vi "Block DMA.vi"(4 "RFM offset":u32 format="%.0x", 6 "Transfer Size (bytes)":u32=1024000, 7 "Wait Mode":T1, 8 "error in (no error)":errorcluster, 11 "VISA Resource Name":refnum<visa-resource-name>="PXI4::14::INSTR") -> (0 "error out":errorcluster, 1 "Read Timed Out?":bool, 2 "Write Timed Out?":bool, 3 "Success?":bool)   [LabVIEW 2017]
uses:
  niveristand-data-sharing-framework-custom-device-plugins/Components/Transceivers/GE Reflective Memory/Driver/Source/Typedefs/GE 5565PIORC.Typedef.DMA Wait Mode.ctl
  niveristand-data-sharing-framework-custom-device-plugins/Components/Transceivers/GE Reflective Memory/Driver/Source/GE 5565PIORC.lvclass/GE 5565PIORC.ctl
  niveristand-data-sharing-framework-custom-device-plugins/Components/Transceivers/GE Reflective Memory/Driver/Source/Methods/GE 5565PIORC.DMA.Block.Write (String).vi
  niveristand-data-sharing-framework-custom-device-plugins/Components/Transceivers/GE Reflective Memory/Driver/Source/Methods/GE 5565PIORC.DMA.Create Transfer (Block).vi
  niveristand-data-sharing-framework-custom-device-plugins/Components/Transceivers/GE Reflective Memory/Driver/Source/Methods/GE 5565PIORC.DMA.Get Transfer Components (Block).vi
  niveristand-data-sharing-framework-custom-device-plugins/Components/Transceivers/GE Reflective Memory/Driver/Source/Methods/GE 5565PIORC.DMA.Block.Read (String).vi
  niveristand-data-sharing-framework-custom-device-plugins/Components/Transceivers/GE Reflective Memory/Driver/Source/Properties/Registers/GE 5565PIORC.Registers.LAS1RR.PCI Address Range.Get.vi
  niveristand-data-sharing-framework-custom-device-plugins/Components/Transceivers/GE Reflective Memory/Driver/Source/Methods/GE 5565PIORC.PXI Interrupts.Enable.vi
  niveristand-data-sharing-framework-custom-device-plugins/Components/Transceivers/GE Reflective Memory/Driver/Source/Properties/Registers/GE 5565PIORC.Registers.DMACSR0.Channel 0 Enable.Set.vi
  niveristand-data-sharing-framework-custom-device-plugins/Components/Transceivers/GE Reflective Memory/Driver/Source/Properties/Registers/GE 5565PIORC.Registers.INTCSR.Local DMA Channel 0 Interrupt Enable.Set.vi
  niveristand-data-sharing-framework-custom-device-plugins/Components/Transceivers/GE Reflective Memory/Driver/Source/Properties/GE 5565PIORC.Read VISA MEMACC.vi
  niveristand-data-sharing-framework-custom-device-plugins/Components/Transceivers/GE Reflective Memory/Driver/Source/Methods/GE 5565PIORC.DMA.Create Transfer (Scatter-Gather).vi
  niveristand-data-sharing-framework-custom-device-plugins/Components/Transceivers/GE Reflective Memory/Driver/Source/Methods/GE 5565PIORC.DMA.Configure.vi
  niveristand-data-sharing-framework-custom-device-plugins/Components/Transceivers/GE Reflective Memory/Driver/Source/Methods/GE 5565PIORC.PXI Interrupts.Discard Events.vi
  niveristand-data-sharing-framework-custom-device-plugins/Components/Transceivers/GE Reflective Memory/Driver/Source/Methods/GE 5565PIORC.DMA.Start.vi
  niveristand-data-sharing-framework-custom-device-plugins/Components/Transceivers/GE Reflective Memory/Driver/Source/Methods/GE 5565PIORC.DMA.Wait for Done.vi
  niveristand-data-sharing-framework-custom-device-plugins/Components/Transceivers/GE Reflective Memory/Driver/Source/Methods/GE 5565PIORC.DMA.Block.Clear.vi
  niveristand-data-sharing-framework-custom-device-plugins/Components/Transceivers/GE Reflective Memory/Driver/Source/Methods/GE 5565PIORC.DMA.Block.Clear (multiple).vi
  niveristand-data-sharing-framework-custom-device-plugins/Components/Transceivers/GE Reflective Memory/Driver/Source/Properties/Registers/GE 5565PIORC.Registers.Local Configuration.Read.vi
  niveristand-data-sharing-framework-custom-device-plugins/Components/Transceivers/GE Reflective Memory/Driver/Source/Properties/Registers/GE 5565PIORC.Registers.Local Configuration.Read (U32).vi
  niveristand-data-sharing-framework-custom-device-plugins/Components/Transceivers/GE Reflective Memory/Driver/Source/Properties/Registers/GE 5565PIORC.Registers.Local Configuration.Read (U8).vi
  niveristand-data-sharing-framework-custom-device-plugins/Components/Transceivers/GE Reflective Memory/Driver/Source/Properties/Registers/GE 5565PIORC.Registers.Local Configuration.Write.vi
  niveristand-data-sharing-framework-custom-device-plugins/Components/Transceivers/GE Reflective Memory/Driver/Source/Properties/Registers/GE 5565PIORC.Registers.Local Configuration.Write (U8).vi
  niveristand-data-sharing-framework-custom-device-plugins/Components/Transceivers/GE Reflective Memory/Driver/Source/Methods/GE 5565PIORC.Bit Manipulation.Set Bit.vi
  niveristand-data-sharing-framework-custom-device-plugins/Components/Transceivers/GE Reflective Memory/Driver/Source/Methods/GE 5565PIORC.Bit Manipulation.Set Bit (U8).vi
  niveristand-data-sharing-framework-custom-device-plugins/Components/Transceivers/GE Reflective Memory/Driver/Source/Properties/Registers/GE 5565PIORC.Registers.Local Configuration.Write (U32).vi
  niveristand-data-sharing-framework-custom-device-plugins/Components/Transceivers/GE Reflective Memory/Driver/Source/Methods/GE 5565PIORC.Bit Manipulation.Set Bit (U32).vi
  niveristand-data-sharing-framework-custom-device-plugins/Components/Transceivers/GE Reflective Memory/Driver/Source/Methods/GE 5565PIORC.DMA.Size.vi
  niveristand-data-sharing-framework-custom-device-plugins/Components/Transceivers/GE Reflective Memory/Driver/Source/Properties/Registers/GE 5565PIORC.Registers.DMADPR0.Direction of Transfer.Set.vi
  niveristand-data-sharing-framework-custom-device-plugins/Components/Transceivers/GE Reflective Memory/Driver/Source/Properties/Registers/GE 5565PIORC.Registers.DMASIZ0.DMA Transfer Size.Set.vi
  niveristand-data-sharing-framework-custom-device-plugins/Components/Transceivers/GE Reflective Memory/Driver/Source/Properties/Registers/GE 5565PIORC.Registers.DMALADR0.Local Address Register.Set.vi
  niveristand-data-sharing-framework-custom-device-plugins/Components/Transceivers/GE Reflective Memory/Driver/Source/Properties/Registers/GE 5565PIORC.Registers.DMAMODE0.Scatter-Gather Mode.Set.vi
  niveristand-data-sharing-framework-custom-device-plugins/Components/Transceivers/GE Reflective Memory/Driver/Source/Properties/Registers/GE 5565PIORC.Registers.DMAPADR0.PCI Address Register.Set.vi
  niveristand-data-sharing-framework-custom-device-plugins/Components/Transceivers/GE Reflective Memory/Driver/Source/Methods/GE 5565PIORC.DMA.Scatter-Gather.Link Block Descriptors.vi
  niveristand-data-sharing-framework-custom-device-plugins/Components/Transceivers/GE Reflective Memory/Driver/Source/Methods/GE 5565PIORC.DMA.Scatter-Gather.Commit Linked Block Descriptors.vi
  niveristand-data-sharing-framework-custom-device-plugins/Components/Transceivers/GE Reflective Memory/Driver/Source/Properties/Registers/GE 5565PIORC.Registers.DMADPR0.Channel 0 First Descriptor Address.Set.vi
  niveristand-data-sharing-framework-custom-device-plugins/Components/Transceivers/GE Reflective Memory/Driver/Source/Methods/GE 5565PIORC.DMA.Get Transfer Components (Scatter-Gather).vi
  <vilib>/Utility/error.llb/Clear Errors.vi
  niveristand-data-sharing-framework-custom-device-plugins/Components/Transceivers/GE Reflective Memory/Driver/Source/Properties/Registers/GE 5565PIORC.Registers.DMACSR0.Channel 0 Start.Set.vi
  niveristand-data-sharing-framework-custom-device-plugins/Components/Transceivers/GE Reflective Memory/Driver/Source/Properties/Registers/GE 5565PIORC.Registers.DMACSR0.Channel 0 Clear Interrupt.Set.vi
  niveristand-data-sharing-framework-custom-device-plugins/Components/Transceivers/GE Reflective Memory/Driver/Source/Methods/GE 5565PIORC.DMA.Poll for Done Signal.vi
  niveristand-data-sharing-framework-custom-device-plugins/Components/Transceivers/GE Reflective Memory/Driver/Source/Methods/GE 5565PIORC.PXI Interrupts.Wait for Event.vi
  niveristand-data-sharing-framework-custom-device-plugins/Components/Transceivers/GE Reflective Memory/Driver/Source/Methods/GE 5565PIORC.DMA.Block.Clear (single).vi
  niveristand-data-sharing-framework-custom-device-plugins/Components/Transceivers/GE Reflective Memory/Driver/Source/Methods/GE 5565PIORC.Registers.Read.vi
  niveristand-data-sharing-framework-custom-device-plugins/Components/Transceivers/GE Reflective Memory/Driver/Source/Methods/GE 5565PIORC.Registers.Read (U32).vi
  niveristand-data-sharing-framework-custom-device-plugins/Components/Transceivers/GE Reflective Memory/Driver/Source/Methods/GE 5565PIORC.Registers.Read (U8).vi
  niveristand-data-sharing-framework-custom-device-plugins/Components/Transceivers/GE Reflective Memory/Driver/Source/Methods/GE 5565PIORC.Registers.Write.vi
  niveristand-data-sharing-framework-custom-device-plugins/Components/Transceivers/GE Reflective Memory/Driver/Source/Methods/GE 5565PIORC.Registers.Write (U8).vi
  niveristand-data-sharing-framework-custom-device-plugins/Components/Transceivers/GE Reflective Memory/Driver/Source/Methods/GE 5565PIORC.Registers.Write (U32).vi
  niveristand-data-sharing-framework-custom-device-plugins/Components/Transceivers/GE Reflective Memory/Driver/Source/Methods/GE 5565PIORC.DMA.Scatter-Gather.Set Descriptor Params.vi
  niveristand-data-sharing-framework-custom-device-plugins/Components/Transceivers/GE Reflective Memory/Driver/Source/Methods/GE 5565PIORC.DMA.Is Done.vi
  niveristand-data-sharing-framework-custom-device-plugins/Components/Transceivers/GE Reflective Memory/Driver/Source/Properties/Registers/GE 5565PIORC.Registers.DMACSR0.Channel 0 Inactive.Get.vi
  niveristand-data-sharing-framework-custom-device-plugins/Components/Transceivers/GE Reflective Memory/Driver/Source/Methods/GE 5565PIORC.Bit Manipulation.Get Bit.vi
  niveristand-data-sharing-framework-custom-device-plugins/Components/Transceivers/GE Reflective Memory/Driver/Source/Methods/GE 5565PIORC.Bit Manipulation.Get Bit (U8).vi
  niveristand-data-sharing-framework-custom-device-plugins/Components/Transceivers/GE Reflective Memory/Driver/Source/Methods/GE 5565PIORC.Round Up to Nearest 8.vi
  niveristand-data-sharing-framework-custom-device-plugins/Components/Transceivers/GE Reflective Memory/Driver/Source/Methods/GE 5565PIORC.Round Up to Nearest 16.vi
  niveristand-data-sharing-framework-custom-device-plugins/Components/Transceivers/GE Reflective Memory/Driver/Source/GE 5565PIORC.lvclass
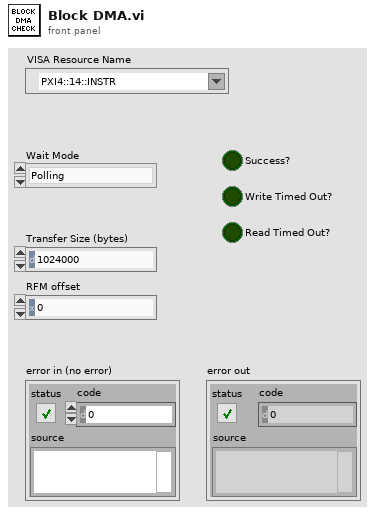
[diagram p1: front panel]
types:
  T1 = typedef "GE 5565PIORC.lvclass/GE 5565PIORC.Typedef.DMA Wait Mode.ctl" = enum16{"Polling", "Interrupt"}
  T2 = typedef "GE 5565PIORC.lvclass/GE 5565PIORC.Typedef.DMA Block Descriptor.ctl" = cluster{"descriptor ptr (VISA)":u32, "descriptor ptr (RFM)":u32, "descriptor size":u32, "descriptor params":T3}
  T3 = typedef "GE 5565PIORC.lvclass/GE 5565PIORC.Typedef.DMA Block Descriptor Params.ctl" = cluster{"data ptr (lower)":u32, "data ptr (upper)":u32, "data size":u32, "next descriptor ptr":u32}
  T4 = typedef "GE 5565PIORC.lvclass/GE 5565PIORC.Typedef.DMA Transfer Spec.ctl" = cluster{"RFM offset":u32, "Block Descriptors":T2[]}
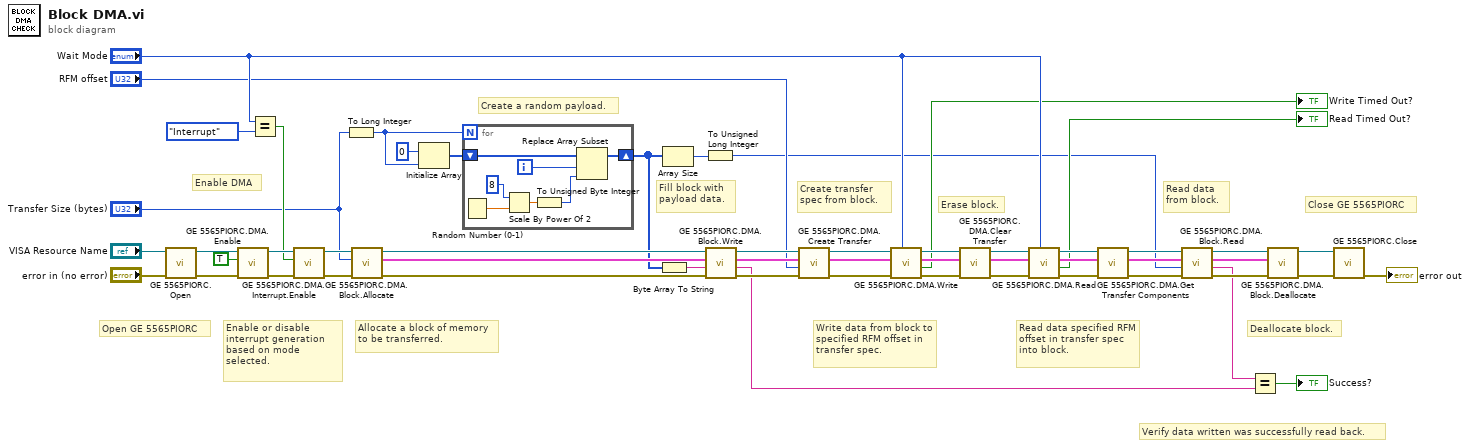
[diagram p0: block diagram]
diagram:
  # "Verify data written was successfully read back."
  # "Close GE 5565PIORC"
  # "Deallocate block."
  # "Erase block."
  # "Read data from block."
  # "Read data specified RFM offset in transfer spec into block."
  # "Write data from block to specified RFM offset in transfer spec."
  # "Create transfer spec from block."
  # "Fill block with payload data."
  # "Allocate a block of memory to be transferred."
  # "Enable or disable interrupt generation based on mode selected."
  # "Enable DMA"
  # "Open GE 5565PIORC"
  # "Create a random payload."
  n1 = call "GE 5565PIORC.Open.vi"("error in (no error)"="error in (no error)", "VISA resource name"="VISA Resource Name") -> ("error out"=w51:errorcluster, "GE 5565PIORC"=w52:refnum<class "GE 5565PIORC.lvclass">)  [unwired: 8 in]
  n2 = call "GE 5565PIORC.DMA.Enable.vi"("error in (no error)"=w51, "enable (T)"=TRUE, "GE 5565PIORC in"=w52) -> ("error out"=w49:errorcluster, "GE 5565PIORC out"=w48:refnum<class "GE 5565PIORC.lvclass">)  [unwired: 7 in]
  n3 = Equal?(x="Wait Mode", y=GE_5565PIORC.Typedef.DMA_Wait_Mode."Interrupt") -> (x = y?=w39:bool)
  n4 = call "GE 5565PIORC.DMA.Interrupt.Enable.vi"("error in (no error)"=w49, "enable (T)"=w39, "GE 5565PIORC in"=w48) -> ("error out"=w45:errorcluster, "GE 5565PIORC out"=w46:refnum<class "GE 5565PIORC.lvclass">)  [unwired: 7 in]
  n5 = To Long Integer(number="Transfer Size (bytes)") -> (32bit integer=w34:i32)
  n6 = call "GE 5565PIORC.DMA.Block.Allocate.vi"("error in (no error)"=w45, "size in bytes"="Transfer Size (bytes)", "GE 5565PIORC in"=w46) -> ("error out"=w27:errorcluster, "Block Descriptor"=w24:T2, "GE 5565PIORC out"=w28:refnum<class "GE 5565PIORC.lvclass">)  [unwired: 6 in]
  n7 = Initialize Array(u8 0, w34) -> (w43:u8[])
  n8 = for {
    N: w34 -> [_]
    shift-right: [w59] -> w20
    shift-left: w43 -> [w60]
    i -> [w58]
    n9 = Random Number (0-1)() -> (number: 0 to 1=w57:dbl)
    n10 = Scale By Power Of 2(n=i16 8, x=w57) -> (x*2^n=w55:dbl)
    n11 = To Unsigned Byte Integer(number=w55) -> (unsigned 8bit integer=w54:u8)
    n12 = Replace Array Subset(array=w60, new element=w54, index=w58) -> (w59:u8[])
  }
  n13 = Byte Array To String(unsigned byte array=w20) -> (string=w21:string)
  n14 = Array Size(array=w20) -> (size(s)=w6:i32)
  n15 = To Unsigned Long Integer(number=w6) -> (unsigned 32bit integer=w3:u32)
  n16 = call-poly "GE 5565PIORC.DMA.Block.Write.vi"("error in (no error)"=w27, "data"=w21, "Block Descriptor in"=w24, "GE 5565PIORC in"=w28) -> ("error out"=w25:errorcluster, "data out"=w22:string, "Block Descriptor out"=w23:T2, "GE 5565PIORC out"=w26:refnum<class "GE 5565PIORC.lvclass">)  [unwired: 4 in]
  n17 = call-poly "GE 5565PIORC.DMA.Create Transfer.vi"("error in (no error)"=w25, "RFM offset"="RFM offset", "Block Descriptor"=w23, "GE 5565PIORC in"=w26) -> ("error out"=w40:errorcluster, "DMA Transfer Spec"=w41:T4, "GE 5565PIORC out"=w42:refnum<class "GE 5565PIORC.lvclass">)  [unwired: 4 in, 1 out]
  n18 = call "GE 5565PIORC.DMA.Write.vi"("wait mode (polling)"="Wait Mode", "error in (no error)"=w40, "DMA Transfer Spec"=w41, "GE 5565PIORC in"=w42) -> ("error out"=w18:errorcluster, "timed out?"=→"Write Timed Out?":bool, "DMA Transfer Spec dup"=w17:T4, "GE 5565PIORC out"=w19:refnum<class "GE 5565PIORC.lvclass">)  [unwired: 4 in]
  n19 = call "GE 5565PIORC.DMA.Clear Transfer.vi"("error in (no error)"=w18, "DMA Transfer Spec in"=w17, "GE 5565PIORC in"=w19) -> ("error out"=w15:errorcluster, "DMA Transfer Spec out"=w14:T4, "GE 5565PIORC out"=w16:refnum<class "GE 5565PIORC.lvclass">)  [unwired: 6 in]
  n20 = call "GE 5565PIORC.DMA.Read.vi"("wait mode (polling)"="Wait Mode", "error in (no error)"=w15, "DMA Transfer Spec"=w14, "GE 5565PIORC in"=w16) -> ("error out"=w11:errorcluster, "timed out?"=→"Read Timed Out?":bool, "DMA Transfer Spec dup"=w10:T4, "GE 5565PIORC out"=w12:refnum<class "GE 5565PIORC.lvclass">)  [unwired: 4 in]
  n21 = call-poly "GE 5565PIORC.DMA.Get Transfer Components.vi"("error in (no error)"=w11, "DMA Transfer Spec in"=w10, "GE 5565PIORC in"=w12) -> ("error out"=w7:errorcluster, "Block Descriptor"=w8:T2, "GE 5565PIORC out"=w9:refnum<class "GE 5565PIORC.lvclass">)  [unwired: 5 in, 1 out]
  n22 = call-poly "GE 5565PIORC.DMA.Block.Read.vi"("error in (no error)"=w7, "bytes to read"=w3, "Block Descriptor in"=w8, "GE 5565PIORC in"=w9) -> ("error out"=w31:errorcluster, "data"=w29:string, "Block Descriptor out"=w30:T2, "GE 5565PIORC out"=w32:refnum<class "GE 5565PIORC.lvclass">)  [unwired: 4 in]
  n23 = Equal?(x=w29, y=w22) -> (x = y?=→"Success?":bool)
  n24 = call "GE 5565PIORC.DMA.Block.Deallocate.vi"("error in (no error)"=w31, "Block Descriptor"=w30, "GE 5565PIORC in"=w32) -> ("error out"=w36:errorcluster, "GE 5565PIORC out"=w37:refnum<class "GE 5565PIORC.lvclass">)  [unwired: 7 in]
  n25 = call "GE 5565PIORC.Close.vi"("error in (no error)"=w36, "GE 5565PIORC in"=w37) -> ("error out"=→"error out":errorcluster)  [unwired: 8 in, 1 out]
